vi "LockIn_#3_data.vi"(1 "Choose Lock-In #3":u16(ring) items=["SR830", "PE7265", "LIA7230", "zurichInst"]) -> (0 "String":string)   [LabVIEW 2019]
uses:
  Instrument_Setup.vi
  Global Variables/Data_Display_global.vi
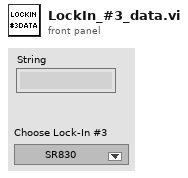
[diagram p1: front panel]
types:
  T1 = typedef "SR830-Settings-Cluster.ctl" = cluster{"VISA":refnum<visa-resource-name>, "Display Channel 2":cluster{" display":i32, " ratio":u16, "output":u16}, "Display Channel 1":cluster{" display":i32, " ratio":u16, "output":u16}, "Time constant":cluster{"time constant\n(10 µs : 0) ":i32, "slope (6 dB/oct)":i32}, "Sensitivity":cluster{"sensitivity\n2nV/fA":i32, "dyn reserve\n(low noise:2)":i16, "ref. phase":ext, "automeasure":bool}, "Offset - Expand.":cluster{"Manual Offset (0)":dbl, "Offset/Expand Parameter (1: X)":u16, "Expand (0: x1)":u16, "Auto Offset ":bool}, "Reference":cluster{"ref. source":bool, "osc.harm# ":u16, "osc. freq":ext, "osc. ampl.":ext, "ref. trigger":u16}, "Lock In 1 sync":cluster{"sync filter":bool, "line filter\n(off:0)":i32}, "Lock In 1 input":cluster{"input":u16, "ground":bool, "couple":bool}}
  T2 = typedef "SR830-Cluster.ctl" = cluster{"Lockin 1":dbl[][], "X1-Display":dbl, "Y1-Display":dbl, "X1 Percent":dbl, "X1 Overload":bool, "Y1 Overload":bool, "Unit X1":string, "Unit X2":string, "Unit X2a":string, "Unit X1a":string, "Sensitivity Setpoint":i16, "X1 Percent 2":dbl, "Y1":dbl, "X1":dbl, "Preamp OVL":bool}
  T3 = typedef "PE7265-Cluster.ctl" = cluster{"Lockin 1":dbl[][], "X1-Display":dbl, "X1 Percent":dbl, "Y1-Display":dbl, "X1 Percent 2":dbl, "Unit X1":string, "Unit X1a":string, "Unit X2":string, "Unit X2a":string, "X1 Overload":bool, "Y1 Overload":bool, "Sensitivity Setpoint":i16, "X1":dbl, "Y1":dbl}
  T4 = cluster{"PE7265 AutoSens at ech step":bool, "PE7265 Sens":i32, "Coupling":bool, "AC Gain":u16, "Auto AC Gain":bool, "Input Device (Voltage Mode)":bool, "Line Frequency":bool, "Input Connector Shells":bool, "PE7265 Input Mode":u16, "Line Frequency\nRejection Filter":u8, "Port":u16, "7265 GPIB Address":i8, "Interface":bool, "Exit":bool, "GPIB Parameter 7260":cluster{"address":string, "delay time":dbl, "mode":i32}, "PE7265 delay after AS":dbl, "VISA session PE7265":refnum<visa-resource-name>, "Slope":u8, "Synchronous TC":bool, "Time Constant":u16, "Reference I/P":u8, "Reference\nHarmonic":u16, "Oscillator Amplitude (Volts rms)":dbl, "Oscillator Frequency (Hz)":dbl, "Ref Unlocked":bool, "Virtual Reference\nMode":bool}
  T5 = typedef "LIA7230-cluster.ctl" = cluster{"Lockin 1":dbl[][], "X1-Display":dbl, "X1 Percent":dbl, "Y1-Display":dbl, "X1 Percent 2":dbl, "Unit X1":string, "Unit X2":string, "X1 Overload":bool, "Y1 Overload":bool, "Sensitivity Setpoint":i16, "X1":dbl, "Y1":dbl, "Channel 3":dbl, "Channel 4":dbl, "Channel 4 Percent":dbl, "Channel 3 Percent ":dbl, "Unit Channel 3":string, "Unit Channel 4":string, "Overload channel 3":bool, "Overload channel 4":bool, "Offsets (ON)":bool, "Sensitivity Setpoint 2":i16}
  T6 = cluster{"Interface":u16, "Port":u16, "Serial Number":string, "IP Address":string, "Line Frequency\nRejection Filter":u8, "Input Mode":u16, "Input Conn. Shells":bool, "Line Frequency":bool, "Auto AC Gain":bool, "AC Gain":u16, "Input Device":bool, "Range":u8, " Auto Sensitivity ":bool, "Auto Measure":bool, "Range 2":u8, " Auto Sensitivity  2":bool, "Slope":u8, "Synchronous TC":bool, "Time Constant":u16, "Slope 2":u8, "Time Constant 2":u16, "Oscillator Amp (V rms)":dbl, "Oscillator Freq (Hz)":dbl, "Reference I/P":u8, "Ref Harm 1":u16, "Ref Harm2":u16, "Virtual Ref.\nMode":bool, "Dual Harmonic/Reference Mode":bool, "Reference Mode":bool, "TRIG OUT\n= Ref Mon":bool, " Auto Phase ":bool, "Reference Phase 1":dbl, "+90 degrees 1":bool, " Auto Phase 2 ":bool, "Reference 2 Phase":dbl, "+90 degrees2":bool, "Auxiliary I/O":bool, "Configuration":bool, "Curve Buffer":bool, "Offsets":bool, "X Channel Offset (%)":sgl, "X Channel Offset":bool, "Y Channel Offset (%)":dbl, "Y Channel Offset":bool, " Auto Offset":bool, "X Channel Offset (%) 2":sgl, "X Channel Offset 2":bool, "Y Channel Offset (%) 2":dbl, "Y Channel Offset 2":bool, " Auto Offset 2":bool, "Display Type channel 1":u16, "Display Type channel 2":u16, "Display Type channel 3":u16, "Display Type channel 4":u16, "Osc Sweeps":bool, "Define Equation1":bool, "Coupling":bool}
  T7 = typedef "Control 3.ctl" = cluster{"Adress":string, "Load Settings from File":bool, "Output_Demod1":enum16{"Aux 1", "Aux 2", "Aux 3", "Aux 4"}, "Input_Demod1":enum16{"Sig In 1", "Curr In 1", "Trigger 1", "Trigger 2", "Aux Out 1", "Aux Out 2", "Aux Out 3", "Aux Out 4", "Aux In 1", "Aux In 2", "Constant"}, "Input_Mode_Demod1":enum16{"single ended", "differential"}, "Bandwith_Mode_Demod1":enum16{"TC", "BW NEP", "BW 3dB"}, "Bandw_Value_demod1":dbl, "Demod1_Range":dbl, "Demod1_Harmonic":dbl, "Trigger_Demod1":enum16{"Manual", "External"}, "osc1_freq":dbl, "osc1_amp":dbl, "Demod1_scaling":dbl, "osc2_freq":dbl, "osc2_amp":dbl, "osc3_freq":dbl, "osc3_amp":dbl, "osc4_freq":dbl, "osc4_amp":dbl, "Demod1_Phase (deg)":dbl, "Demod1_order":ext, "Demod1_coupling":enum16{"DC", "AC"}, "Demod1_shields":enum16{"Ground", "Float"}, "Demod1_input_resistance":enum16{"10M", "50"}, "Demod1_Ref_oscillator":ext, "Demod1_output_imp":enum16{"Disable", "Enable"}, "Demod1_output_diff":enum16{"Disable", "Enable"}, "Demod1_rate":dbl, "Demod1_Output_range":dbl, "Output_Demod2":enum16{"Aux 1", "Aux 2", "Aux 3", "Aux 4"}, "Demod2_input":enum16{"Sig In 1", "Curr In 1", "Trigger 1", "Trigger 2", "Aux Out 1", "Aux Out 2", "Aux Out 3", "Aux Out 4", "Aux In 1", "Aux In 2", "Constant"}, "Input_Mode_Demod2":enum16{"single ended", "differential"}, "Bandwith_Mode_Demod2":enum16{"TC", "BW NEP", "BW 3dB"}, "Bandw_Value_demod2":dbl, "Demod2_Range":dbl, "Demod2_Harmonic":dbl, "Trigger_Demod2":enum16{"Manual", "External"}, "Demod2_scaling":dbl, "Demod2_Phase (deg)":dbl, "Demod2_order":ext, "Demod2_coupling":enum16{"DC", "AC"}, "Demod2_shields":enum16{"Ground", "Float"}, "Demod2_input_resistance":enum16{"10M", "50"}, "Demod2_Ref_oscillator":ext, "Demod2_output_imp":enum16{"Disable", "Enable"}, "Demod2_output_diff":enum16{"Disable", "Enable"}, "Demod2_rate":dbl, "Demod2_Output_range":dbl, "Output_Demod3":enum16{"Aux 1", "Aux 2", "Aux 3", "Aux 4"}, "Demod3_input":enum16{"Sig In 1", "Curr In 1", "Trigger 1", "Trigger 2", "Aux Out 1", "Aux Out 2", "Aux Out 3", "Aux Out 4", "Aux In 1", "Aux In 2", "Constant"}, "Input_Mode_Demod3":enum16{"single ended", "differential"}, "Bandwith_Mode_Demod2":enum16{"TC", "BW NEP", "BW 3dB"}, "Bandw_Value_demod3":dbl, "Demod3_Range":dbl, "Demod3_Harmonic":dbl, "Trigger_Demod3":enum16{"Manual", "External"}, "Demod3_scaling":dbl, "Demod3_Phase (deg)":dbl, "Demod3_order":ext, "Demod3_coupling":enum16{"DC", "AC"}, "Demod3_shields":enum16{"Ground", "Float"}, "Demod3_input_resistance":enum16{"10M", "50"}, "Demod3_Ref_oscillator":ext, "Demod3_output_imp":enum16{"Disable", "Enable"}, "Demod3_output_diff":enum16{"Disable", "Enable"}, "Demod3_rate":dbl, "Demod3_Output_range":dbl, "Output_Demod4":enum16{"Aux 1", "Aux 2", "Aux 3", "Aux 4"}, "Demod4_input":enum16{"Sig In 1", "Curr In 1", "Trigger 1", "Trigger 2", "Aux Out 1", "Aux Out 2", "Aux Out 3", "Aux Out 4", "Aux In 1", "Aux In 2", "Constant"}, "Input_Mode_Demod4":enum16{"single ended", "differential"}, "Bandwith_Mode_Demod4":enum16{"TC", "BW NEP", "BW 3dB"}, "Bandw_Value_demod4":dbl, "Demod4_Range":dbl, "Demod4_Harmonic":dbl, "Trigger_Demod4":enum16{"Manual", "External"}, "Demod4_scaling":dbl, "Demod4_Phase (deg)":dbl, "Demod4_order":ext, "Demod4_coupling":enum16{"DC", "AC"}, "Demod4_shields":enum16{"Ground", "Float"}, "Demod4_input_resistance":enum16{"10M", "50"}, "Demod4_Ref_oscillator":ext, "Demod4_output_imp":enum16{"Disable", "Enable"}, "Demod4_output_diff":enum16{"Disable", "Enable"}, "Demod4_rate":dbl, "Demod4_Output_range":dbl, "Oscillator1_Amp_units":enum16{"Vpk", "Vrms", "VdBm"}, "Oscillator4_Amp_units":enum16{"Vpk", "Vrms", "VdBm"}, "Oscillator2_Amp_units":enum16{"Vpk", "Vrms", "VdBm"}, "Oscillator3_Amp_units":enum16{"Vpk", "Vrms", "VdBm"}, "Demod1_sync_filter":enum16{"Disable", "Enable"}, "Demod 1 (on/off)":bool, "Demod 2 (on/off) ":bool, "Demod 3 (on/off) ":bool, "Demod 4 (on/off) ":bool, " Sigouts 1 (on/off)":bool, " Sigouts 2 (on/off) ":bool, " Sigouts 3 (on/off)":bool, " Sigouts 4 (on/off) ":bool, "Demod2_sync_filter":enum16{"Disable", "Enable"}, "Demod1_auto_outp_rang":enum16{"Disable", "Enable"}, "Demod2_auto_outp_rang ":enum16{"Disable", "Enable"}}
  T8 = typedef "MFLIMonitor_Cluster.ctl" = cluster{"Demod 0":dbl[][], " Demod 1":dbl[][], "Demod 0 :X":dbl, "Demod 0 :Y ":dbl, "Demod 1 :X":dbl, "Demod 1 :Y ":dbl, " Demod 2":dbl[][], "Demod 3":dbl[][], "Demod 2 :X":dbl, "Demod 2 :Y ":dbl, "Demod 3 :X ":dbl, "Demod 3 :Y ":dbl, "Demod Sample out 0 ":T9, "Demod Sample out 1":T9, "Demod Sample out 2":T9, "Demod Sample out 3":T9, "Update Lock-In":bool, "Connected ?":bool, "Demod 0 Zero Phase":bool, "Demod 1 Zero Phase":bool, "Demod 2 Zero Phase":bool, "Demod 3 Zero Phase":bool, "Osc 0 Freq":dbl, "Osc 1 Freq":dbl, "Osc 2 Freq":dbl, "Osc 3 Freq":dbl, "Clipping":bool, "Range (V)":dbl, "Offset (V)":dbl, "Auto-Range":bool, "Add":bool, "Diff":bool, "On":bool, "50 Ohm":bool, "Ampl 0 Enable":bool, "Ampl 1 Enable":bool, "Ampl 2 Enable":bool, "Ampl 3 Enable":bool, "Ampl 0":dbl, "Ampl 1":dbl, "Ampl 2":dbl, "Ampl 3":dbl, "Update Osci":bool, "Output Range (V) ":dbl, "Set Range (in)":bool}
  T9 = typedef "Zurich Instruments LabOne.lvlib/ziTypeDemodSampleEx.ctl" = cluster{"Timestamps (ticks)":u64[], "X (Vrms)":dbl[], "Y (Vrms)":dbl[], "Osc Phase (rad)":dbl[], "Freq (Hz)":dbl[], "DIO":u32[], "Aux In 0 (V)":dbl[], "Aux In 1 (V)":dbl[], "Trigger":u32[]}
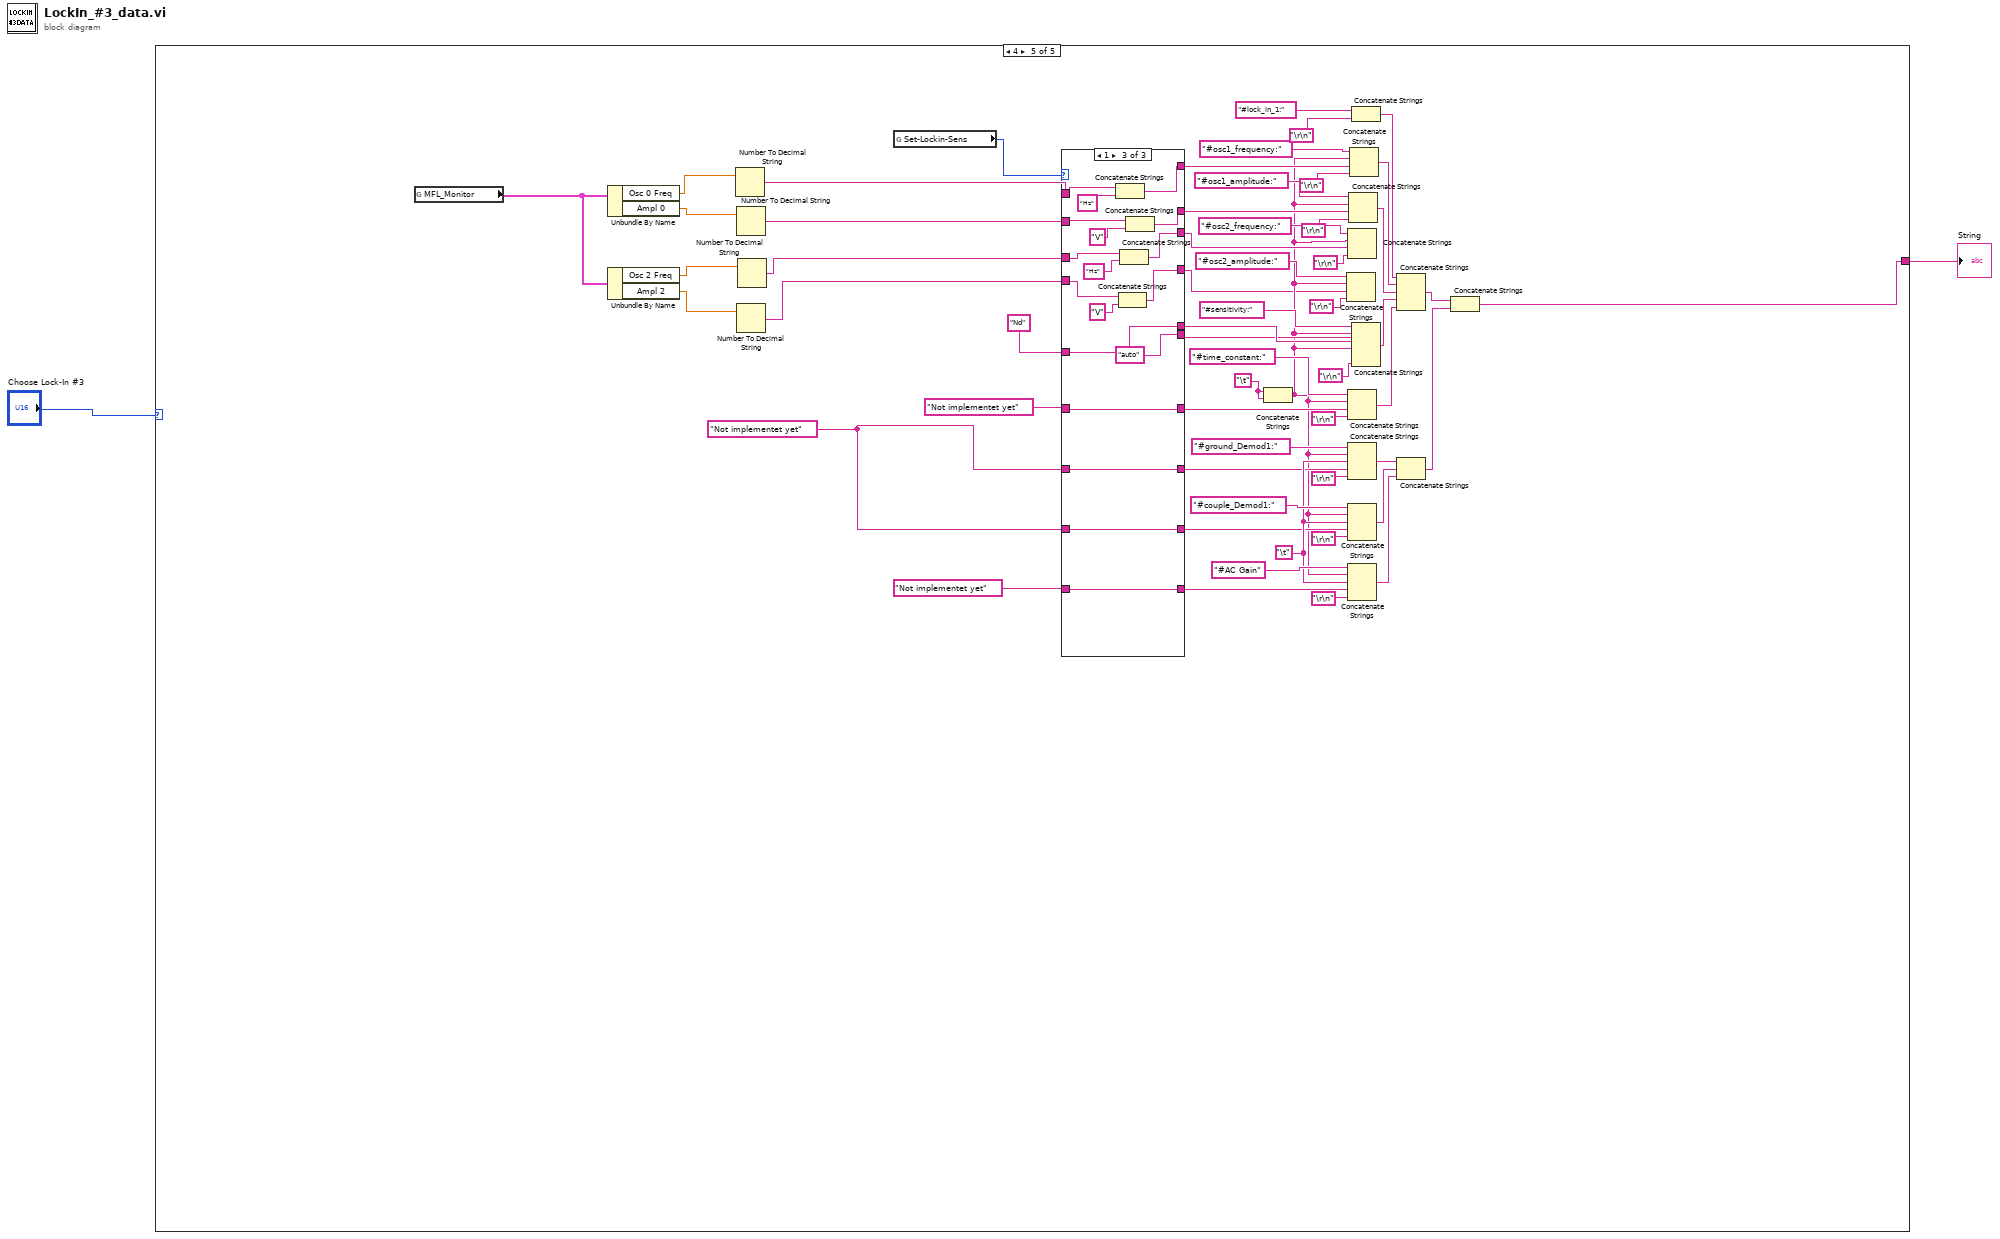
[diagram p0: block diagram]
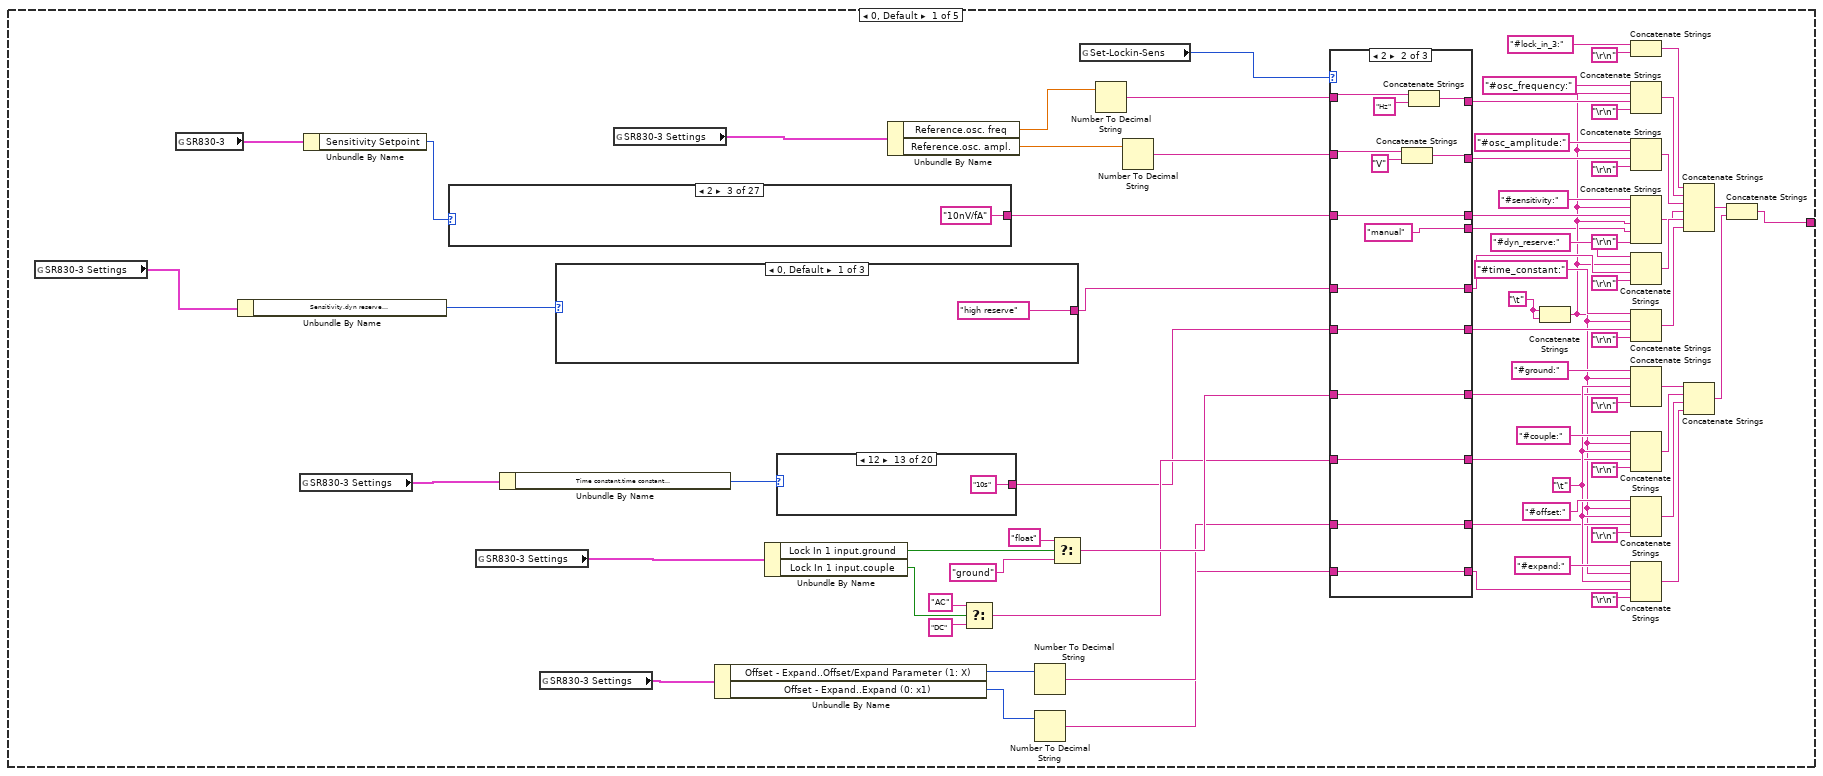
[diagram p2: hidden frame]
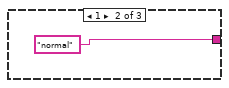
[diagram p3: hidden frame]
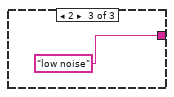
[diagram p4: hidden frame]
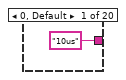
[diagram p5: hidden frame]
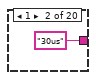
[diagram p6: hidden frame]
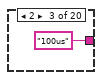
[diagram p7: hidden frame]
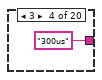
[diagram p8: hidden frame]
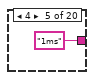
[diagram p9: hidden frame]
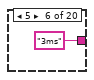
[diagram p10: hidden frame]
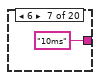
[diagram p11: hidden frame]
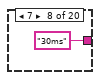
[diagram p12: hidden frame]
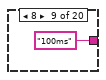
[diagram p13: hidden frame]
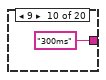
[diagram p14: hidden frame]
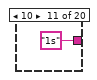
[diagram p15: hidden frame]
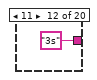
[diagram p16: hidden frame]
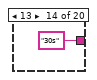
[diagram p17: hidden frame]
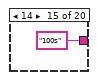
[diagram p18: hidden frame]
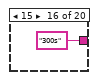
[diagram p19: hidden frame]
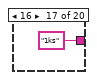
[diagram p20: hidden frame]
diagram:
  n1 = case shown="4" "Choose Lock-In #3" {
    tunnel: [w3 w230 w335 w716 w835] -> w2
    frame 0, Default {
      w36 = "\t"
      w77 = "\t"
      n2 = global read "Instrument_Setup.vi" "SR830-3 Settings"() -> (w43:T1)
      n3 = global read "Data_Display_global.vi" "SR830-3"() -> (w7:T2)
      n4 = Unbundle By Name(w43) -> ("Sensitivity.dyn reserve\n(low noise:2)"=w9:i16)
      n5 = global read "Instrument_Setup.vi" "SR830-3 Settings"() -> (w49:T1)
      n6 = Unbundle By Name(w7) -> ("Sensitivity Setpoint"=w6:i16)
      n7 = case shown="2" w6 {
        tunnel: ["2nV/fA" "5nV/fA" "10nV/fA" "20nV/fA" "50nV/fA" "100nV/fA" "200nV/fA" "500nV/fA" "1uV/pA" "2uV/pA" "5uV/pA" "10uV/pA" "20uV/pA" "50uV/pA" "100uV/pA" "200uV/pA" "500uV/pA" "1mV/nA" "2mV/nA" "5mV/nA" "10mV/nA" "20mV/nA" "50mV/nA" "100mV/nA" "200mV/nA" "500mV/nA" "1V/uA"] -> w13
        frame 0, Default {
        }
        frame 1 {
        }
        frame 2 {
        }
        frame 3 {
        }
        frame 4 {
        }
        frame 5 {
        }
        frame 6 {
        }
        frame 7 {
        }
        frame 8 {
        }
        frame 9 {
        }
        frame 10 {
        }
        frame 11 {
        }
        frame 12 {
        }
        frame 13 {
        }
        frame 14 {
        }
        frame 15 {
        }
        frame 16 {
        }
        frame 17 {
        }
        frame 18 {
        }
        frame 19 {
        }
        frame 20 {
        }
        frame 21 {
        }
        frame 22 {
        }
        frame 23 {
        }
        frame 24 {
        }
        frame 25 {
        }
        frame 26 {
        }
      }
      n8 = global read "Instrument_Setup.vi" "SR830-3 Settings"() -> (w55:T1)
      n9 = Unbundle By Name(w49) -> ("Time constant.time constant\n(10 µs : 0)"=w12:i32)
      n10 = global read "Instrument_Setup.vi" "SR830-3 Settings"() -> (w62:T1)
      n11 = case shown="0, Default" w9 {
        tunnel: ["high reserve" "normal" "low noise"] -> w10
        frame 0, Default {
        }
        frame 1 {
        }
        frame 2 {
        }
      }
      n12 = global read "Instrument_Setup.vi" "SR830-3 Settings"() -> (w41:T1)
      n13 = Unbundle By Name(w62) -> ("Offset - Expand..Offset/Expand Parameter (1: X)"=w33:u16, "Offset - Expand..Expand (0: x1)"=w32:u16)
      n14 = Unbundle By Name(w55) -> ("Lock In 1 input.ground"=w56:bool, "Lock In 1 input.couple"=w30:bool)
      n15 = case shown="12" w12 {
        tunnel: ["10us" "30us" "100us" "300us" "1ms" "3ms" "10ms" "30ms" "100ms" "300ms" "1s" "3s" "10s" "30s" "100s" "300s" "1ks" "3ks" "10ks" "30ks"] -> w11
        frame 0, Default {
        }
        frame 1 {
        }
        frame 2 {
        }
        frame 3 {
        }
        frame 4 {
        }
        frame 5 {
        }
        frame 6 {
        }
        frame 7 {
        }
        frame 8 {
        }
        frame 9 {
        }
        frame 10 {
        }
        frame 11 {
        }
        frame 12 {
        }
        frame 13 {
        }
        frame 14 {
        }
        frame 15 {
        }
        frame 16 {
        }
        frame 17 {
        }
        frame 18 {
        }
        frame 19 {
        }
      }
      n16 = Unbundle By Name(w41) -> ("Reference.osc. freq"=w35:ext, "Reference.osc. ampl."=w34:ext)
      n17 = Select(t="AC", s=w30, f="DC") -> (s? t:f=w25:string)
      n18 = Number To Decimal String(number=w33) -> (decimal integer string=w23:string)  [unwired: 1 in]
      n19 = Number To Decimal String(number=w32) -> (decimal integer string=w21:string)  [unwired: 1 in]
      n20 = Select(t="float", s=w56, f="ground") -> (s? t:f=w27:string)
      n21 = global read "Instrument_Setup.vi" "Set-Lockin-Sens"() -> (w29:u16)
      n22 = Number To Decimal String(number=w35) -> (decimal integer string=w19:string)  [unwired: 1 in]
      n23 = Number To Decimal String(number=w34) -> (decimal integer string=w17:string)  [unwired: 1 in]
      n24 = case shown="2" w29 {
        tunnel: w11 -> [w129 w149 w163]
        tunnel: [w129 w149 w163] -> w28
        tunnel: w27 -> [w141 w155 w169]
        tunnel: [w141 w155 w169] -> w26
        tunnel: w25 -> [w140 w154 w168]
        tunnel: [w140 w154 w168] -> w24
        tunnel: [w138 w152 w166] -> w22
        tunnel: w23 -> [w138 w152 w166]
        tunnel: w21 -> [w139 w153 w167]
        tunnel: [w139 w153 w167] -> w20
        tunnel: w19 -> [w136 w145 w159]
        tunnel: [w135 w143 w157] -> w18
        tunnel: w17 -> [w133 w144 w158]
        tunnel: [w132 w142 w156] -> w16
        tunnel: w13 -> [w131 w151 w165]
        tunnel: [w131 w151 w165] -> w15
        tunnel: w10 -> [w130 w150 w164]
        tunnel: [w130 w150 w164] -> w14
        tunnel: ["Command-file" "manual" "auto"] -> w4
        frame 0, Default {
          n25 = Concatenate Strings(w133, "V" ("String")) -> (w132:string)
          n26 = Concatenate Strings(w136, "Hz" ("String")) -> (w135:string)
        }
        frame 2 {
          n27 = Concatenate Strings(w144, "V" ("String")) -> (w142:string)
          n28 = Concatenate Strings(w145, "Hz" ("String")) -> (w143:string)
        }
        frame 1 {
          n29 = Concatenate Strings(w158, "V" ("String")) -> (w156:string)
          n30 = Concatenate Strings(w159, "Hz" ("String")) -> (w157:string)
        }
      }
      n31 = Concatenate Strings(w77, w77) -> (w5:string)
      n32 = Concatenate Strings("#lock_in_3:", "\r\n") -> (w40:string)
      n33 = Concatenate Strings("#osc_frequency:", w5, w18, "\r\n") -> (w66:string)
      n34 = Concatenate Strings("#osc_amplitude:" ("String"), w5, w16, "\r\n") -> (w67:string)
      n35 = Concatenate Strings("#sensitivity:" ("String"), w5, w15, w5, w4, "\r\n") -> (w68:string)
      n36 = Concatenate Strings("#dyn_reserve:" ("String"), w5, w14, "\r\n") -> (w69:string)
      n37 = Concatenate Strings("#time_constant:" ("String"), w5, w28, "\r\n") -> (w70:string)
      n38 = Concatenate Strings("#ground:" ("String"), w5, w36, w26, "\r\n") -> (w71:string)
      n39 = Concatenate Strings("#couple:" ("String"), w5, w36, w24, "\r\n") -> (w72:string)
      n40 = Concatenate Strings("#offset:" ("String"), w5, w36, w22, "\r\n") -> (w73:string)
      n41 = Concatenate Strings("#expand:" ("String"), w5, w36, w20, "\r\n") -> (w74:string)
      n42 = Concatenate Strings(w40, w66, w67, w68, w69, w70) -> (w75:string)
      n43 = Concatenate Strings(w71, w72, w73, w74) -> (w76:string)
      n44 = Concatenate Strings(w75, w76) -> (w3:string)
    }
    frame 1 {
      w197 = "\t"
      w231 = "\t"
      n45 = global read "Data_Display_global.vi" "PE7265-Cluster"() -> (w176:T3)
      n46 = Unbundle By Name(w176) -> ("Sensitivity Setpoint"=w175:i16)
      n47 = global read "Instrument_Setup.vi" "PE7625-Settings-3"() -> (w206:T4)
      n48 = case shown="2" w175 {
        tunnel: ["2nV/fA" "5nV/fA" "10nV/fA" "20nV/fA" "50nV/fA" "100nV/fA" "200nV/fA" "500nV/fA" "1uV/pA" "2uV/pA" "5uV/pA" "10uV/pA" "20uV/pA" "50uV/pA" "100uV/pA" "200uV/pA" "500uV/pA" "1mV/nA" "2mV/nA" "5mV/nA" "10mV/nA" "20mV/nA" "50mV/nA" "100mV/nA" "200mV/nA" "500mV/nA" "1V/uA"] -> w180
        frame 0, Default {
        }
        frame 1 {
        }
        frame 2 {
        }
        frame 3 {
        }
        frame 4 {
        }
        frame 5 {
        }
        frame 6 {
        }
        frame 7 {
        }
        frame 8 {
        }
        frame 9 {
        }
        frame 10 {
        }
        frame 11 {
        }
        frame 12 {
        }
        frame 13 {
        }
        frame 14 {
        }
        frame 15 {
        }
        frame 16 {
        }
        frame 17 {
        }
        frame 18 {
        }
        frame 19 {
        }
        frame 20 {
        }
        frame 21 {
        }
        frame 22 {
        }
        frame 23 {
        }
        frame 24 {
        }
        frame 25 {
        }
        frame 26 {
        }
      }
      n49 = global read "Instrument_Setup.vi" "PE7625-Settings-3"() -> (w212:T4)
      n50 = global read "Instrument_Setup.vi" "PE7625-Settings-3"() -> (w219:T4)
      n51 = Unbundle By Name(w206) -> ("Time Constant"=w179:u16)
      n52 = global read "Instrument_Setup.vi" "PE7625-Settings-3"() -> (w201:T4)
      n53 = Unbundle By Name(w219) -> ("AC Gain"=w171:u16)
      n54 = Unbundle By Name(w212) -> ("Input Connector Shells"=w213:bool, "Coupling"=w193:bool)
      n55 = case shown="0, Default" w179 {
        tunnel: ["10us" "20us" "40us" "80us" "160us" "320us" "640us" "5ms" "10ms" "20ms" "50ms" "100ms" "200ms" "500ms" "1s" "2s" "5s" "10s" "20s" "50s" "100s" "200s" "500s" "1ks" "2ks" "5ks" "10ks" "20ks" "50ks" "100ks"] -> w178
        frame 0, Default {
        }
        frame 1 {
        }
        frame 2 {
        }
        frame 3 {
        }
        frame 4 {
        }
        frame 5 {
        }
        frame 6 {
        }
        frame 7 {
        }
        frame 8 {
        }
        frame 9 {
        }
        frame 10 {
        }
        frame 11 {
        }
        frame 12 {
        }
        frame 13 {
        }
        frame 14 {
        }
        frame 15 {
        }
        frame 16 {
        }
        frame 17 {
        }
        frame 18 {
        }
        frame 19 {
        }
        frame 20 {
        }
        frame 21 {
        }
        frame 22 {
        }
        frame 23 {
        }
        frame 24 {
        }
        frame 25 {
        }
        frame 26 {
        }
        frame 27 {
        }
        frame 28 {
        }
        frame 29 {
        }
      }
      n56 = Unbundle By Name(w201) -> ("Oscillator Frequency (Hz)"=w196:dbl, "Oscillator Amplitude (Volts rms)"=w195:dbl)
      n57 = case shown="9" w171 {
        tunnel: ["0dB" "10dB" "20dB" "30dB" "40dB" "50dB" "60dB" "70dB" "80dB" "90dB"] -> w170
        frame 0, Default {
        }
        frame 1 {
        }
        frame 2 {
        }
        frame 3 {
        }
        frame 4 {
        }
        frame 5 {
        }
        frame 6 {
        }
        frame 7 {
        }
        frame 8 {
        }
        frame 9 {
        }
      }
      n58 = Select(t="DC", s=w193, f="AC") -> (s? t:f=w188:string)
      n59 = Select(t="float", s=w213, f="ground") -> (s? t:f=w190:string)
      n60 = global read "Instrument_Setup.vi" "Set-Lockin-Sens"() -> (w192:u16)
      n61 = Number To Decimal String(number=w196) -> (decimal integer string=w185:string)  [unwired: 1 in]
      n62 = Number To Decimal String(number=w195) -> (decimal integer string=w183:string)  [unwired: 1 in]
      n63 = case shown="1" w192 {
        tunnel: w178 -> [w300 w318 w330]
        tunnel: [w300 w318 w330] -> w191
        tunnel: w190 -> [w310 w322 w334]
        tunnel: [w310 w322 w334] -> w189
        tunnel: w188 -> [w309 w321 w333]
        tunnel: [w309 w321 w333] -> w187
        tunnel: [w308 w320 w332] -> w186
        tunnel: w170 -> [w308 w320 w332]
        tunnel: w185 -> [w306 w314 w326]
        tunnel: [w305 w312 w324] -> w184
        tunnel: w183 -> [w303 w313 w325]
        tunnel: [w302 w311 w323] -> w182
        tunnel: w180 -> [w301 w319 w331]
        tunnel: [w301 w319 w331] -> w181
        tunnel: ["Command-file" "manual" "auto"] -> w173
        frame 0, Default {
          n64 = Concatenate Strings(w303, "V" ("String")) -> (w302:string)
          n65 = Concatenate Strings(w306, "Hz" ("String")) -> (w305:string)
        }
        frame 2 {
          n66 = Concatenate Strings(w313, "V" ("String")) -> (w311:string)
          n67 = Concatenate Strings(w314, "Hz" ("String")) -> (w312:string)
        }
        frame 1 {
          n68 = Concatenate Strings(w325, "V" ("String")) -> (w323:string)
          n69 = Concatenate Strings(w326, "Hz" ("String")) -> (w324:string)
        }
      }
      n70 = Concatenate Strings(w231, w231) -> (w174:string)
      n71 = Concatenate Strings("#lock_in_3:", "\r\n") -> (w200:string)
      n72 = Concatenate Strings("#osc_frequency:", w174, w184, "\r\n") -> (w222:string)
      n73 = Concatenate Strings("#osc_amplitude:" ("String"), w174, w182, "\r\n") -> (w223:string)
      n74 = Concatenate Strings("#sensitivity:" ("String"), w174, w181, w174, w173, "\r\n") -> (w224:string)
      n75 = Concatenate Strings("#time_constant:" ("String"), w174, w191, "\r\n") -> (w172:string)
      n76 = Concatenate Strings("#ground:" ("String"), w174, w197, w189, "\r\n") -> (w225:string)
      n77 = Concatenate Strings("#couple:" ("String"), w174, w197, w187, "\r\n") -> (w226:string)
      n78 = Concatenate Strings("#AC Gain" ("String"), w174, w197, w186, "\r\n") -> (w227:string)
      n79 = Concatenate Strings(w200, w222, w223, w224, w172) -> (w228:string)
      n80 = Concatenate Strings(w225, w226, w227) -> (w229:string)
      n81 = Concatenate Strings(w228, w229) -> (w230:string)
    }
    frame 2 {
      w354 = "\t"
      w364 = "\t"
      w458 = "\t"
      n82 = global read "Data_Display_global.vi" "LIA7230-Cluster-3"() -> (w397:T5)
      n83 = global read "Instrument_Setup.vi" "LIA7230-Setup-Custer 3"() -> (w389:T6)
      n84 = Unbundle By Name(w397) -> ("Sensitivity Setpoint 2"=w396:i16)
      n85 = Unbundle By Name(w397) -> ("Sensitivity Setpoint"=w399:i16)
      n86 = global read "Instrument_Setup.vi" "LIA7230-Setup-Custer 3"() -> (w361:T6)
      n87 = case shown="0" w399 {
        tunnel: ["N/A" "2nV/fA" "5nV/fA" "10nV/fA" "20nV/fA" "50nV/fA" "100nV/fA" "200nV/fA" "500nV/fA" "1uV/pA" "2uV/pA" "5uV/pA" "10uV/pA" "20uV/pA" "50uV/pA" "100uV/pA" "200uV/pA" "500uV/pA" "1mV/nA" "2mV/nA" "5mV/nA" "10mV/nA" "20mV/nA" "50mV/nA" "100mV/nA" "200mV/nA" "500mV/nA" "1V/uA"] -> w403
        frame 0 {
        }
        frame 1, Default {
        }
        frame 2 {
        }
        frame 3 {
        }
        frame 4 {
        }
        frame 5 {
        }
        frame 6 {
        }
        frame 7 {
        }
        frame 8 {
        }
        frame 9 {
        }
        frame 10 {
        }
        frame 11 {
        }
        frame 12 {
        }
        frame 13 {
        }
        frame 14 {
        }
        frame 15 {
        }
        frame 16 {
        }
        frame 17 {
        }
        frame 18 {
        }
        frame 19 {
        }
        frame 20 {
        }
        frame 21 {
        }
        frame 22 {
        }
        frame 23 {
        }
        frame 24 {
        }
        frame 25 {
        }
        frame 26 {
        }
        frame 27 {
        }
      }
      n88 = global read "Instrument_Setup.vi" "LIA7230-Setup-Custer 3"() -> (w439:T6)
      n89 = case shown="0" w396 {
        tunnel: ["N/A" "2nV/fA" "5nV/fA" "10nV/fA" "20nV/fA" "50nV/fA" "100nV/fA" "200nV/fA" "500nV/fA" "1uV/pA" "2uV/pA" "5uV/pA" "10uV/pA" "20uV/pA" "50uV/pA" "100uV/pA" "200uV/pA" "500uV/pA" "1mV/nA" "2mV/nA" "5mV/nA" "10mV/nA" "20mV/nA" "50mV/nA" "100mV/nA" "200mV/nA" "500mV/nA" "1V/uA"] -> w395
        frame 0 {
        }
        frame 1, Default {
        }
        frame 2 {
        }
        frame 3 {
        }
        frame 4 {
        }
        frame 5 {
        }
        frame 6 {
        }
        frame 7 {
        }
        frame 8 {
        }
        frame 9 {
        }
        frame 10 {
        }
        frame 11 {
        }
        frame 12 {
        }
        frame 13 {
        }
        frame 14 {
        }
        frame 15 {
        }
        frame 16 {
        }
        frame 17 {
        }
        frame 18 {
        }
        frame 19 {
        }
        frame 20 {
        }
        frame 21 {
        }
        frame 22 {
        }
        frame 23 {
        }
        frame 24 {
        }
        frame 25 {
        }
        frame 26 {
        }
        frame 27 {
        }
      }
      n90 = Unbundle By Name(w389) -> ("Time Constant 2"=w388:u16)
      n91 = Unbundle By Name(w389) -> ("Time Constant"=w402:u16)
      n92 = Unbundle By Name(w361) -> ("Display Type channel 4"=w337:u16)
      n93 = Unbundle By Name(w361) -> ("Display Type channel 1"=w362:u16)
      n94 = Unbundle By Name(w361) -> ("Display Type channel 3"=w359:u16)
      n95 = Unbundle By Name(w361) -> ("Display Type channel 2"=w360:u16)
      n96 = global read "Instrument_Setup.vi" "LIA7230-Setup-Custer 3"() -> (w429:T6)
      n97 = case shown="22" w362 {
        tunnel: ["X%" "Y%" "X Calibrated" "Y Calibrated" "Mag %" "Mag Calibrated" "Phase Degree" "Ratio" "Log Ratio" "ADC 1" "ADC 2" "ADC 3" "ADC 4" "Noise %" "Noise Calibrated" "Ref Frequency" "Equation 1" "Equation 2" "X2 %" "Y2 %" "Mag2 %" "Mag2 Calibrated" "Phase2 Degrees"] -> w358
        frame 0, Default {
        }
        frame 1 {
        }
        frame 2 {
        }
        frame 3 {
        }
        frame 4 {
        }
        frame 5 {
        }
        frame 6 {
        }
        frame 7 {
        }
        frame 8 {
        }
        frame 9 {
        }
        frame 10 {
        }
        frame 11 {
        }
        frame 12 {
        }
        frame 13 {
        }
        frame 14 {
        }
        frame 15 {
        }
        frame 16 {
        }
        frame 17 {
        }
        frame 18 {
        }
        frame 19 {
        }
        frame 20 {
        }
        frame 21 {
        }
        frame 22 {
        }
      }
      n98 = case shown="22" w360 {
        tunnel: ["X%" "Y%" "X Calibrated" "Y Calibrated" "Mag %" "Mag Calibrated" "Phase Degree" "Ratio" "Log Ratio" "ADC 1" "ADC 2" "ADC 3" "ADC 4" "Noise %" "Noise Calibrated" "Ref Frequency" "Equation 1" "Equation 2" "X2 %" "Y2 %" "Mag2 %" "Mag2 Calibrated" "Phase2 Degrees"] -> w357
        frame 0, Default {
        }
        frame 1 {
        }
        frame 2 {
        }
        frame 3 {
        }
        frame 4 {
        }
        frame 5 {
        }
        frame 6 {
        }
        frame 7 {
        }
        frame 8 {
        }
        frame 9 {
        }
        frame 10 {
        }
        frame 11 {
        }
        frame 12 {
        }
        frame 13 {
        }
        frame 14 {
        }
        frame 15 {
        }
        frame 16 {
        }
        frame 17 {
        }
        frame 18 {
        }
        frame 19 {
        }
        frame 20 {
        }
        frame 21 {
        }
        frame 22 {
        }
      }
      n99 = Unbundle By Name(w439) -> ("Input Conn. Shells"=w440:bool, "Line Frequency"=w419:bool)
      n100 = case shown="22" w359 {
        tunnel: ["X%" "Y%" "X Calibrated" "Y Calibrated" "Mag %" "Mag Calibrated" "Phase Degree" "Ratio" "Log Ratio" "ADC 1" "ADC 2" "ADC 3" "ADC 4" "Noise %" "Noise Calibrated" "Ref Frequency" "Equation 1" "Equation 2" "X2 %" "Y2 %" "Mag2 %" "Mag2 Calibrated" "Phase2 Degrees"] -> w356
        frame 0, Default {
        }
        frame 1 {
        }
        frame 2 {
        }
        frame 3 {
        }
        frame 4 {
        }
        frame 5 {
        }
        frame 6 {
        }
        frame 7 {
        }
        frame 8 {
        }
        frame 9 {
        }
        frame 10 {
        }
        frame 11 {
        }
        frame 12 {
        }
        frame 13 {
        }
        frame 14 {
        }
        frame 15 {
        }
        frame 16 {
        }
        frame 17 {
        }
        frame 18 {
        }
        frame 19 {
        }
        frame 20 {
        }
        frame 21 {
        }
        frame 22 {
        }
      }
      n101 = Unbundle By Name(w361) -> ("X Channel Offset (%) 2"=w381:sgl, "Y Channel Offset (%) 2"=w377:dbl)
      n102 = Unbundle By Name(w361) -> ("X Channel Offset (%)"=w422:sgl, "Y Channel Offset (%)"=w421:dbl)
      n103 = case shown="12" w388 {
        tunnel: ["10us" "30us" "100us" "300us" "1ms" "3ms" "10ms" "30ms" "100ms" "300ms" "1s" "3s" "10s" "30s" "100s" "300s" "1ks" "3ks" "10ks" "30ks"] -> w387
        frame 0, Default {
        }
        frame 1 {
        }
        frame 2 {
        }
        frame 3 {
        }
        frame 4 {
        }
        frame 5 {
        }
        frame 6 {
        }
        frame 7 {
        }
        frame 8 {
        }
        frame 9 {
        }
        frame 10 {
        }
        frame 11 {
        }
        frame 12 {
        }
        frame 13 {
        }
        frame 14 {
        }
        frame 15 {
        }
        frame 16 {
        }
        frame 17 {
        }
        frame 18 {
        }
        frame 19 {
        }
      }
      n104 = case shown="12" w402 {
        tunnel: ["10us" "30us" "100us" "300us" "1ms" "3ms" "10ms" "30ms" "100ms" "300ms" "1s" "3s" "10s" "30s" "100s" "300s" "1ks" "3ks" "10ks" "30ks"] -> w401
        frame 0, Default {
        }
        frame 1 {
        }
        frame 2 {
        }
        frame 3 {
        }
        frame 4 {
        }
        frame 5 {
        }
        frame 6 {
        }
        frame 7 {
        }
        frame 8 {
        }
        frame 9 {
        }
        frame 10 {
        }
        frame 11 {
        }
        frame 12 {
        }
        frame 13 {
        }
        frame 14 {
        }
        frame 15 {
        }
        frame 16 {
        }
        frame 17 {
        }
        frame 18 {
        }
        frame 19 {
        }
      }
      n105 = case shown="22" w337 {
        tunnel: ["X%" "Y%" "X Calibrated" "Y Calibrated" "Mag %" "Mag Calibrated" "Phase Degree" "Ratio" "Log Ratio" "ADC 1" "ADC 2" "ADC 3" "ADC 4" "Noise %" "Noise Calibrated" "Ref Frequency" "Equation 1" "Equation 2" "X2 %" "Y2 %" "Mag2 %" "Mag2 Calibrated" "Phase2 Degrees"] -> w336
        frame 0, Default {
        }
        frame 1 {
        }
        frame 2 {
        }
        frame 3 {
        }
        frame 4 {
        }
        frame 5 {
        }
        frame 6 {
        }
        frame 7 {
        }
        frame 8 {
        }
        frame 9 {
        }
        frame 10 {
        }
        frame 11 {
        }
        frame 12 {
        }
        frame 13 {
        }
        frame 14 {
        }
        frame 15 {
        }
        frame 16 {
        }
        frame 17 {
        }
        frame 18 {
        }
        frame 19 {
        }
        frame 20 {
        }
        frame 21 {
        }
        frame 22 {
        }
      }
      n106 = Unbundle By Name(w361) -> ("Reference Mode"=w371:bool)
      n107 = Unbundle By Name(w429) -> ("Oscillator Freq (Hz)"=w424:dbl, "Oscillator Amp (V rms)"=w423:dbl)
      n108 = Select(t="50 HZ", s=w419, f="60 Hz") -> (s? t:f=w414:string)
      n109 = Select(t="Dual", s=w371, f="Single") -> (s? t:f=w368:string)
      n110 = Number To Decimal String(number=w377) -> (decimal integer string=w376:string)  [unwired: 1 in]
      n111 = Number To Decimal String(number=w381) -> (decimal integer string=w380:string)  [unwired: 1 in]
      n112 = Number To Decimal String(number=w422) -> (decimal integer string=w412:string)  [unwired: 1 in]
      n113 = Number To Decimal String(number=w421) -> (decimal integer string=w410:string)  [unwired: 1 in]
      n114 = Select(t="float", s=w440, f="ground") -> (s? t:f=w416:string)
      n115 = global read "Instrument_Setup.vi" "Set-Lockin-Sens"() -> (w418:u16)
      n116 = Number To Decimal String(number=w424) -> (decimal integer string=w408:string)  [unwired: 1 in]
      n117 = Number To Decimal String(number=w423) -> (decimal integer string=w406:string)  [unwired: 1 in]
      n118 = case shown="1" w418 {
        tunnel: w401 -> [w655 w678 w701]
        tunnel: [w654 w677 w700] -> w417
        tunnel: w416 -> [w669 w692 w715]
        tunnel: [w669 w692 w715] -> w415
        tunnel: w414 -> [w668 w691 w714]
        tunnel: [w668 w691 w714] -> w413
        tunnel: [w666 w689 w712] -> w411
        tunnel: w412 -> [w666 w689 w712]
        tunnel: w410 -> [w667 w690 w713]
        tunnel: [w667 w690 w713] -> w409
        tunnel: w408 -> [w664 w684 w707]
        tunnel: [w663 w682 w705] -> w407
        tunnel: w406 -> [w661 w683 w706]
        tunnel: [w660 w681 w704] -> w405
        tunnel: w403 -> [w659 w688 w711]
        tunnel: [w659 w688 w711] -> w404
        tunnel: ["Command-file" "manual" "auto"] -> w398
        tunnel: w395 -> [w657 w680 w703]
        tunnel: [w657 w680 w703] -> w392
        tunnel: ["manual" "manual" "manual"] -> w391
        tunnel: w387 -> [w654 w677 w700]
        tunnel: [w655 w678 w701] -> w384
        tunnel: w380 -> [w653 w676 w699]
        tunnel: [w653 w676 w699] -> w379
        tunnel: w376 -> [w652 w675 w698]
        tunnel: [w652 w675 w698] -> w373
        tunnel: w368 -> [w651 w674 w697]
        tunnel: [w651 w674 w697] -> w363
        tunnel: w358 -> [w650 w673 w696]
        tunnel: w357 -> [w649 w672 w695]
        tunnel: w356 -> [w648 w671 w694]
        tunnel: w336 -> [w647 w670 w693]
        tunnel: [w650 w673 w696] -> w353
        tunnel: [w649 w672 w695] -> w350
        tunnel: [w648 w671 w694] -> w347
        tunnel: [w647 w670 w693] -> w343
        frame 0, Default {
          n119 = Concatenate Strings(w661, "V" ("String")) -> (w660:string)
          n120 = Concatenate Strings(w664, "Hz" ("String")) -> (w663:string)
        }
        frame 2 {
          n121 = Concatenate Strings(w683, "V" ("String")) -> (w681:string)
          n122 = Concatenate Strings(w684, "Hz" ("String")) -> (w682:string)
        }
        frame 1 {
          n123 = Concatenate Strings(w706, "V" ("String")) -> (w704:string)
          n124 = Concatenate Strings(w707, "Hz" ("String")) -> (w705:string)
        }
      }
      n125 = Concatenate Strings(w458, w458) -> (w365:string)
      n126 = Concatenate Strings(w354, w354) -> (w344:string)
      n127 = Concatenate Strings("#ground:" ("String"), w365, w364, w415, "\r\n") -> (w452:string)
      n128 = Concatenate Strings("#time_constant2:" ("String"), w365, w417, "\r\n") -> (w390:string)
      n129 = Concatenate Strings("#time_constant1:" ("String"), w365, w384, "\r\n") -> ()  [unwired: 1 out]
      n130 = Concatenate Strings("#sensitivity2:" ("String"), w365, w392, w365, w391, "\r\n") -> ()  [unwired: 1 out]
      n131 = Concatenate Strings("#lock_in_1:", "\r\n") -> (w428:string)
      n132 = Concatenate Strings("#osc_frequency:", w365, w407, "\r\n") -> (w449:string)
      n133 = Concatenate Strings("#osc_amplitude:" ("String"), w365, w405, "\r\n") -> (w450:string)
      n134 = Concatenate Strings("#sensitivity1:" ("String"), w365, w404, w365, w398, "\r\n") -> (w451:string)
      n135 = Concatenate Strings("#Xoffset2:" ("String"), w365, w364, w379, "\r\n") -> (w383:string)
      n136 = Concatenate Strings("#Xoffset:" ("String"), w365, w364, w411, "\r\n") -> (w454:string)
      n137 = Concatenate Strings("#Line Frequency:" ("String"), w365, w364, w413, "\r\n") -> (w453:string)
      n138 = Concatenate Strings("#Yoffset:" ("String"), w365, w364, w409, "\r\n") -> (w455:string)
      n139 = Concatenate Strings("Display Type channel 1:", w344, w353, "\r\n") -> (w341:string)
      n140 = Concatenate Strings("#Yoffset2:" ("String"), w365, w364, w373, "\r\n") -> (w375:string)
      n141 = Concatenate Strings("#Reference Mode:" ("String"), w365, w364, w363, "\r\n") -> ()  [unwired: 1 out]
      n142 = Concatenate Strings("Display Type channel 3:", w344, w347, "\r\n") -> (w339:string)
      n143 = Concatenate Strings("Display Type channel 2:", w344, w350, "\r\n") -> (w340:string)
      n144 = Concatenate Strings("Display Type channel 4:", w344, w343, "\r\n") -> (w338:string)
      n145 = Concatenate Strings(w428, w449, w450, w451, w390) -> (w456:string)
      n146 = Concatenate Strings(w452, w453, w454, w455, w383, w375, w341, w340, w339, w338) -> (w457:string)
      n147 = Concatenate Strings(w456, w457) -> (w335:string)
    }
    frame 3 {
      w752 = "\t"
      w776 = "\t"
      n148 = global read "Instrument_Setup.vi" "zurichInst-1-Settings"() -> (w722:T7)
      n149 = Unbundle By Name(w722) -> ("osc1_freq"=w740:dbl, "osc1_amp"=w738:dbl)
      n150 = Unbundle By Name(w722) -> ("osc2_freq"=w736:dbl, "osc2_amp"=w735:dbl)
      n151 = Unbundle By Name(w722) -> ("Demod1_shields"=w724:enum16{"Ground", "Float"})
      n152 = Unbundle By Name(w722) -> ("Demod1_coupling"=w721:enum16{"DC", "AC"})
      n153 = Number To Decimal String(number=w740) -> (decimal integer string=w739:string)  [unwired: 1 in]
      n154 = Number To Decimal String(number=w738) -> (decimal integer string=w737:string)  [unwired: 1 in]
      n155 = Number To Decimal String(number=w735) -> (decimal integer string=w733:string)  [unwired: 1 in]
      n156 = Number To Decimal String(number=w736) -> (decimal integer string=w734:string)  [unwired: 1 in]
      n157 = case shown="\"Float\"" w724 {
        tunnel: ["Ground" "Float"] -> w723
        frame "Ground", Default {
        }
        frame "Float" {
        }
      }
      n158 = case shown="\"DC\", Default" w721 {
        tunnel: ["DC" "AC"] -> w720
        frame "DC", Default {
        }
        frame "AC" {
        }
      }
      n159 = case shown="2" 1 {
        tunnel: "Not implementet yet" -> [w788 w812 w830]
        tunnel: [w788 w812 w830] -> w751
        tunnel: w723 -> [w798 w816 w834]
        tunnel: [w798 w816 w834] -> w750
        tunnel: w720 -> [w797 w815 w833]
        tunnel: [w797 w815 w833] -> w749
        tunnel: [w796 w814 w832] -> w748
        tunnel: "Not implementet yet" -> [w796 w814 w832]
        tunnel: w739 -> [w794 w808 w826]
        tunnel: [w793 w806 w824] -> w747
        tunnel: w737 -> [w791 w807 w825]
        tunnel: [w790 w805 w823] -> w746
        tunnel: "Nd" -> [w789 w813 w831]
        tunnel: [w789 w813 w831] -> w745
        tunnel: ["Command-file" "manual" "auto"] -> w743
        tunnel: w734 -> [w786 w803 w822]
        tunnel: w733 -> [w785 w802 w820]
        tunnel: [w784 w801 w818] -> w731
        tunnel: [w783 w800 w817] -> w727
        frame 0, Default {
          n160 = Concatenate Strings(w791, "V" ("String")) -> (w790:string)
          n161 = Concatenate Strings(w794, "Hz" ("String")) -> (w793:string)
          n162 = Concatenate Strings(w785, "V" ("String")) -> (w783:string)
          n163 = Concatenate Strings(w786, "Hz" ("String")) -> (w784:string)
        }
        frame 2 {
          n164 = Concatenate Strings(w807, "V" ("String")) -> (w805:string)
          n165 = Concatenate Strings(w802, "V" ("String")) -> (w800:string)
          n166 = Concatenate Strings(w803, "Hz" ("String")) -> (w801:string)
          n167 = Concatenate Strings(w808, "Hz" ("String")) -> (w806:string)
        }
        frame 1 {
          n168 = Concatenate Strings(w826, "Hz" ("String")) -> (w824:string)
          n169 = Concatenate Strings(w820, "V" ("String")) -> (w817:string)
          n170 = Concatenate Strings(w822, "Hz" ("String")) -> (w818:string)
          n171 = Concatenate Strings(w825, "V" ("String")) -> (w823:string)
        }
      }
      n172 = Concatenate Strings(w776, w776) -> (w728:string)
      n173 = Concatenate Strings("#osc2_amplitude:" ("String"), w728, w727, "\r\n") -> ()  [unwired: 1 out]
      n174 = Concatenate Strings("#osc2_frequency:", w728, w731, "\r\n") -> ()  [unwired: 1 out]
      n175 = Concatenate Strings("#time_constant:" ("String"), w728, w751, "\r\n") -> (w717:string)
      n176 = Concatenate Strings("#ground_Demod1:" ("String"), w728, w752, w750, "\r\n") -> (w771:string)
      n177 = Concatenate Strings("#couple_Demod1:" ("String"), w728, w752, w749, "\r\n") -> (w772:string)
      n178 = Concatenate Strings("#AC Gain" ("String"), w728, w752, w748, "\r\n") -> (w773:string)
      n179 = Concatenate Strings("#osc1_amplitude:" ("String"), w728, w746, "\r\n") -> (w770:string)
      n180 = Concatenate Strings("#osc1_frequency:", w728, w747, "\r\n") -> (w769:string)
      n181 = Concatenate Strings("#lock_in_3:", "\r\n") -> (w755:string)
      n182 = Concatenate Strings("#sensitivity:" ("String"), w728, w745, w728, w743, "\r\n") -> (w718:string)
      n183 = Concatenate Strings(w755, w769, w770, w718, w717) -> (w774:string)
      n184 = Concatenate Strings(w771, w772, w773) -> (w775:string)
      n185 = Concatenate Strings(w774, w775) -> (w716:string)
    }
    frame 4 {
      w837 = "Not implementet yet"
      w868 = "\t"
      w892 = "\t"
      n186 = global read "Data_Display_global.vi" "MFL_Monitor"() -> (w836:T8)
      n187 = Unbundle By Name(w836) -> ("Osc 0 Freq"=w857:dbl, "Ampl 0"=w855:dbl)
      n188 = Unbundle By Name(w836) -> ("Osc 2 Freq"=w853:dbl, "Ampl 2"=w852:dbl)
      n189 = Number To Decimal String(number=w857) -> (decimal integer string=w856:string)  [unwired: 1 in]
      n190 = Number To Decimal String(number=w855) -> (decimal integer string=w854:string)  [unwired: 1 in]
      n191 = Number To Decimal String(number=w852) -> (decimal integer string=w850:string)  [unwired: 1 in]
      n192 = Number To Decimal String(number=w853) -> (decimal integer string=w851:string)  [unwired: 1 in]
      n193 = global read "Instrument_Setup.vi" "Set-Lockin-Sens"() -> (w838:u16)
      n194 = case shown="1" w838 {
        tunnel: "Not implementet yet" -> [w900 w924 w942]
        tunnel: [w900 w924 w942] -> w867
        tunnel: w837 -> [w910 w928 w946]
        tunnel: [w910 w928 w946] -> w866
        tunnel: w837 -> [w909 w927 w945]
        tunnel: [w909 w927 w945] -> w865
        tunnel: [w908 w926 w944] -> w864
        tunnel: "Not implementet yet" -> [w908 w926 w944]
        tunnel: w856 -> [w906 w920 w938]
        tunnel: [w905 w918 w936] -> w863
        tunnel: w854 -> [w903 w919 w937]
        tunnel: [w902 w917 w935] -> w862
        tunnel: "Nd" -> [w901 w925 w943]
        tunnel: [w901 w925 w943] -> w861
        tunnel: ["Command-file" "manual" "auto"] -> w859
        tunnel: w851 -> [w898 w915 w934]
        tunnel: w850 -> [w897 w914 w932]
        tunnel: [w896 w913 w930] -> w848
        tunnel: [w895 w912 w929] -> w844
        frame 0, Default {
          n195 = Concatenate Strings(w903, "V" ("String")) -> (w902:string)
          n196 = Concatenate Strings(w906, "Hz" ("String")) -> (w905:string)
          n197 = Concatenate Strings(w897, "V" ("String")) -> (w895:string)
          n198 = Concatenate Strings(w898, "Hz" ("String")) -> (w896:string)
        }
        frame 2 {
          n199 = Concatenate Strings(w919, "V" ("String")) -> (w917:string)
          n200 = Concatenate Strings(w914, "V" ("String")) -> (w912:string)
          n201 = Concatenate Strings(w915, "Hz" ("String")) -> (w913:string)
          n202 = Concatenate Strings(w920, "Hz" ("String")) -> (w918:string)
        }
        frame 1 {
          n203 = Concatenate Strings(w938, "Hz" ("String")) -> (w936:string)
          n204 = Concatenate Strings(w932, "V" ("String")) -> (w929:string)
          n205 = Concatenate Strings(w934, "Hz" ("String")) -> (w930:string)
          n206 = Concatenate Strings(w937, "V" ("String")) -> (w935:string)
        }
      }
      n207 = Concatenate Strings(w892, w892) -> (w845:string)
      n208 = Concatenate Strings("#osc2_amplitude:" ("String"), w845, w844, "\r\n") -> ()  [unwired: 1 out]
      n209 = Concatenate Strings("#osc2_frequency:", w845, w848, "\r\n") -> ()  [unwired: 1 out]
      n210 = Concatenate Strings("#time_constant:" ("String"), w845, w867, "\r\n") -> (w839:string)
      n211 = Concatenate Strings("#ground_Demod1:" ("String"), w845, w868, w866, "\r\n") -> (w887:string)
      n212 = Concatenate Strings("#couple_Demod1:" ("String"), w845, w868, w865, "\r\n") -> (w888:string)
      n213 = Concatenate Strings("#AC Gain" ("String"), w845, w868, w864, "\r\n") -> (w889:string)
      n214 = Concatenate Strings("#osc1_amplitude:" ("String"), w845, w862, "\r\n") -> (w886:string)
      n215 = Concatenate Strings("#osc1_frequency:", w845, w863, "\r\n") -> (w885:string)
      n216 = Concatenate Strings("#lock_in_1:", "\r\n") -> (w871:string)
      n217 = Concatenate Strings("#sensitivity:" ("String"), w845, w861, w845, w859, "\r\n") -> (w840:string)
      n218 = Concatenate Strings(w871, w885, w886, w840, w839) -> (w890:string)
      n219 = Concatenate Strings(w887, w888, w889) -> (w891:string)
      n220 = Concatenate Strings(w890, w891) -> (w835:string)
    }
  }
  "String" <- w2
